vi "Read_binary_data.vi"() -> (0 "Analogue Frequency Hz":dbl format="%.2f", 1 "PWA Binary":i16[][](array[numeric]), 2 "Analogue Binary":i16[][](array[numeric])=[[142, 132, 123, 114, 103, 93, 84, 74, 65, 56, 49, 42, 35, 30, 27, 24, 23, 22, 24, 26, 30, 35, 41, 48, 56, 65, 73, 82, 93, 102, 112, 122, 132, 141, 149, 156, 164, 169, 173, 177, 180, 181, 181, 179, 176, 171, 167, 160, 153, 145, 137, 128, 118, 108, 98, 88, 79, 69, 61, 52, 45, 38, 33, 28, 25, 23, 22, 23, 25, 29, 32, 39, 45, 52, 60, 69, 78, 88, 97, 108, 118, 127, 136, 145, 153, 160, 166, 171, 176, 179, 180, 181, 180, 178, 174, 169, 164, 157, 149, 141]], 3 "PWA Frequency Hz":dbl format="%.2f", 4 "LDA Binary output":u16[][](array[numeric])=[[142, 132, 123, 114, 103, 93, 84, 74, 65, 56, 49, 42, 35, 30, 27, 24, 23, 22, 24, 26, 30, 35, 41, 48, 56, 65, 73, 82, 93, 102, 112, 122, 132, 141, 149, 156, 164, 169, 173, 177, 180, 181, 181, 179, 176, 171, 167, 160, 153, 145, 137, 128, 118, 108, 98, 88, 79, 69, 61, 52, 45, 38, 33, 28, 25, 23, 22, 23, 25, 29, 32, 39, 45, 52, 60, 69, 78, 88, 97, 108, 118, 127, 136, 145, 153, 160, 166, 171, 176, 179, 180, 181, 180, 178, 174, 169, 164, 157, 149, 141]], 5 "EOF?":bool, 6 "Block Header":string)   [LabVIEW 2010]
uses:
  Globals/Meas_global.vi
  Globals/LDA_meas_global_1.vi
panel:
  out "string":string
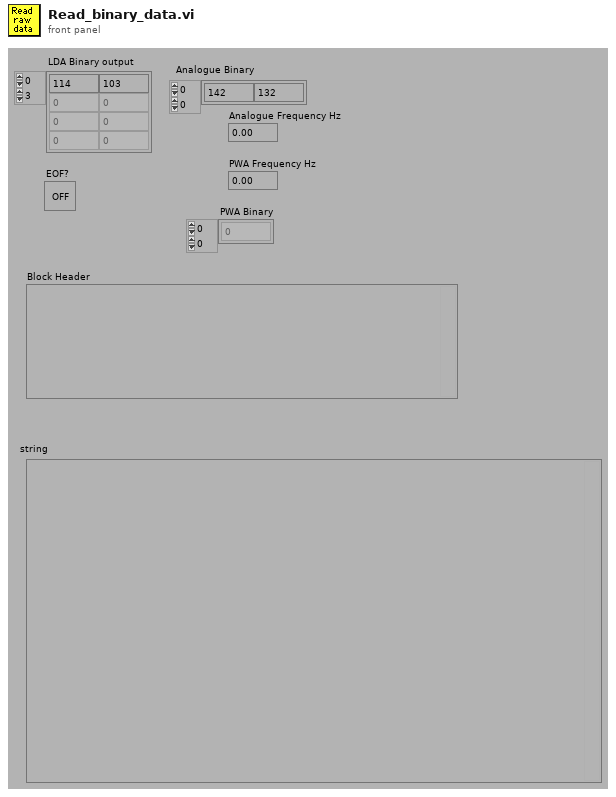
[diagram p1: front panel]
types:
  T1 = enum16{"read/write", "read-only", "write-only", "write-only (truncate)"}
  T2 = typedef "Ch_and_Spans.ctl" = cluster{"high limit (10V)":sgl, "low limit (-10V)":sgl, "Ch No":i16, "Var name":string, "Use Latest Calib":bool}
  T3 = typedef "BSA_Type.ctl" = enum16{"57N11", "BSA F60"}
  T4 = typedef "PWA_Data.ctl" = enum16{"No PWA Data", "One Ch PWA"}
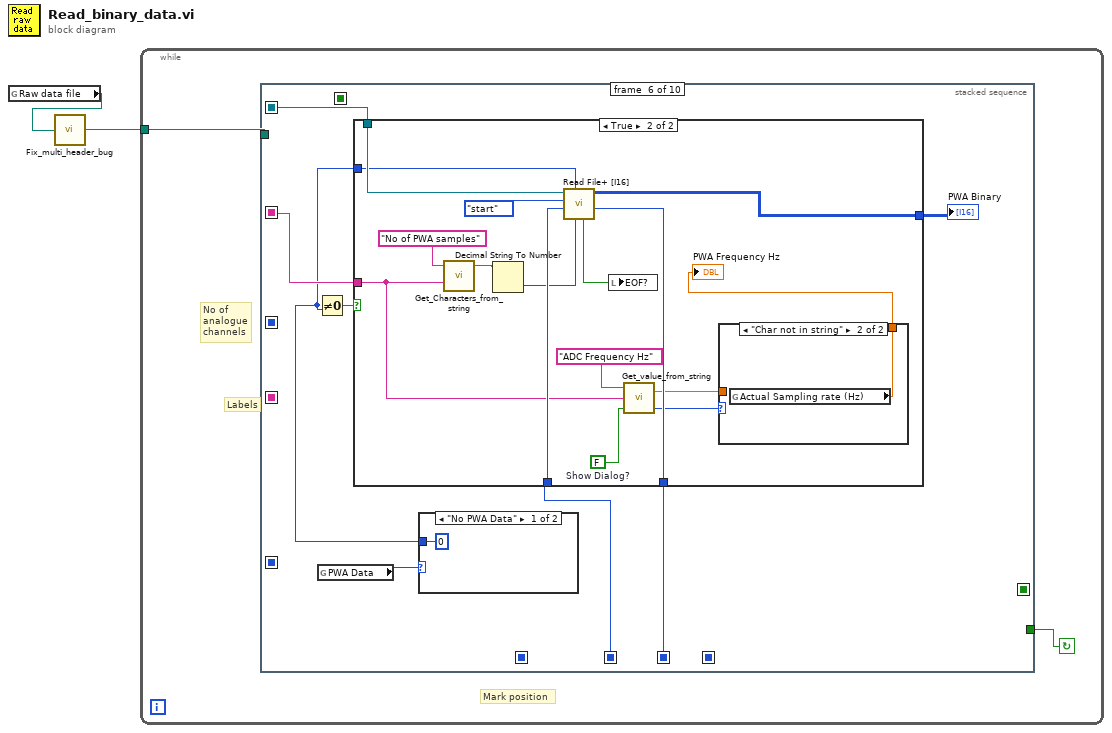
[diagram p0: block diagram]
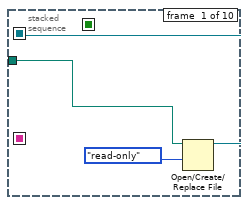
[diagram p2: hidden frame]
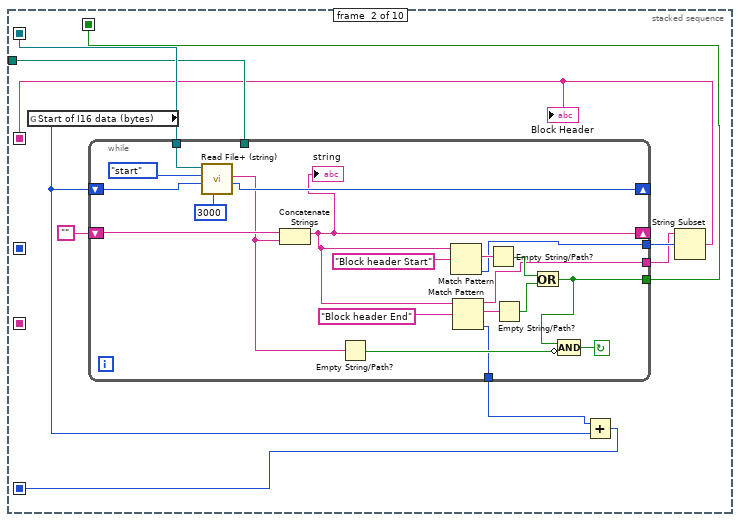
[diagram p3: hidden frame]
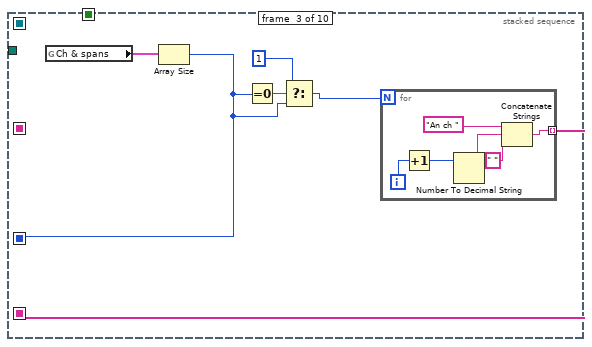
[diagram p4: hidden frame]
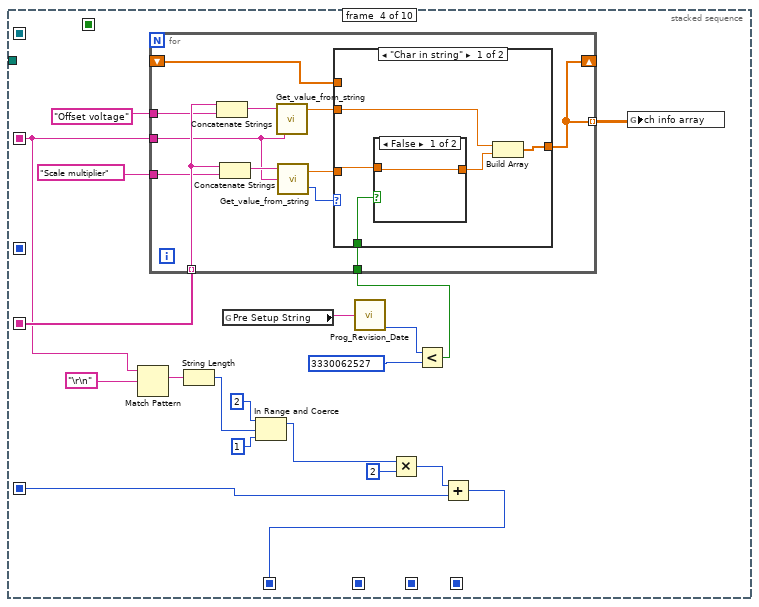
[diagram p5: hidden frame]
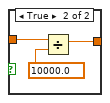
[diagram p6: hidden frame]
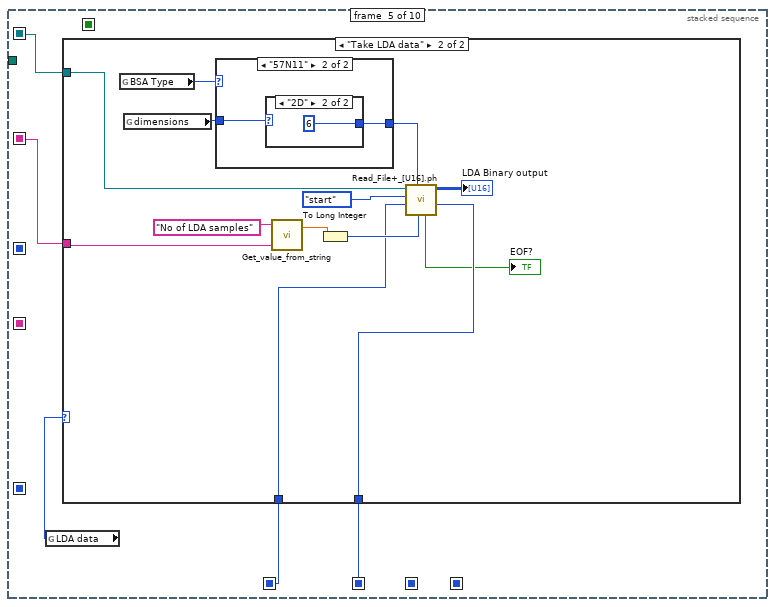
[diagram p8: hidden frame]
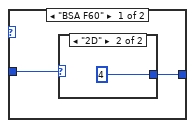
[diagram p10: hidden frame]
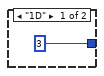
[diagram p11: hidden frame]
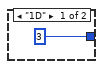
[diagram p12: hidden frame]
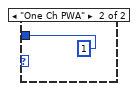
[diagram p13: hidden frame]
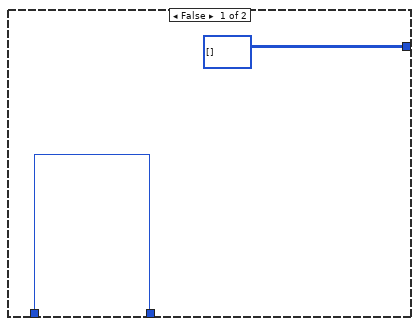
[diagram p14: hidden frame]
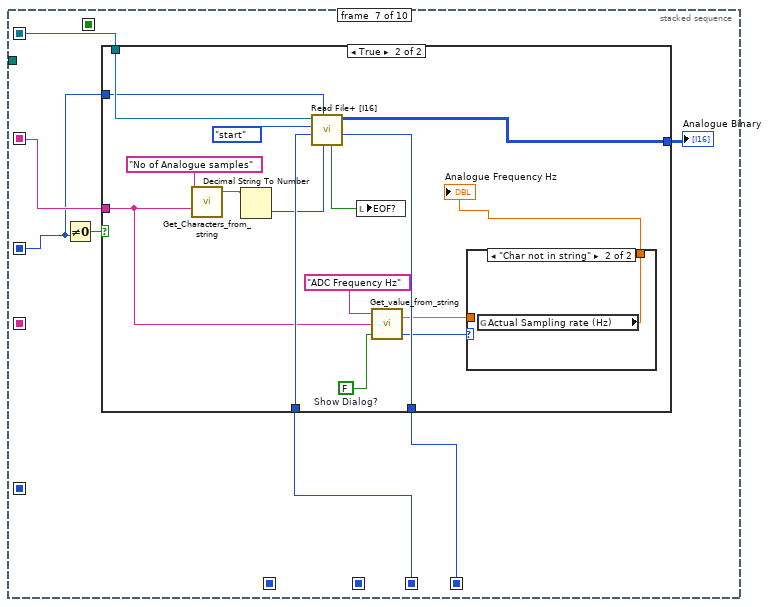
[diagram p16: hidden frame]
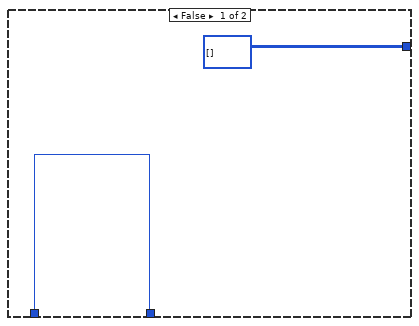
[diagram p17: hidden frame]
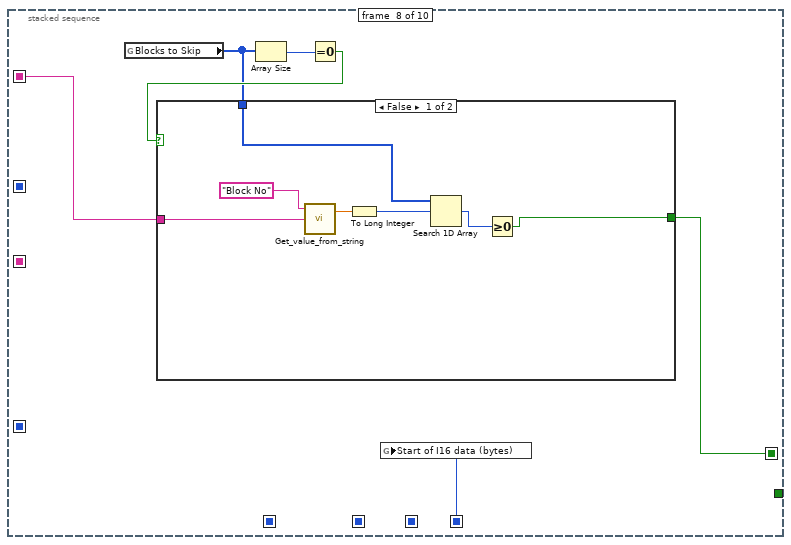
[diagram p19: hidden frame]
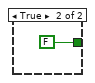
[diagram p20: hidden frame]
diagram:
  n1 = global read "Meas_global.vi" "Raw data file"() -> (w2:path)
  n2 = call "Fix_multi_header_bug.vi"("Raw data File to Read"=w2) -> ("Raw data File to Read Out"=w1:path)
  n3 = while {
    tunnel: w1 -> [w4]
    stop <- w3 continue-if-true
    # "Mark position"
    # "Labels"
    # "No of\nanalogue\nchannels"
    n4 = stacked-sequence {
      seq-local: [w6 _ _ _ _ _ _ _ _ _] -> [_ w17 _ _ w91 w122 w153 _ w194 w213]
      seq-local: [_ w8 _ _ _ _ _ _ _ _] -> [_ _ _ w55 w94 w125 w154 w178 _ _]
      seq-local: [_ _ w40 _ _ _ _ _ _ _] -> [_ _ _ _ _ _ w151 _ _ _]
      seq-local: [_ _ w42 _ _ _ _ _ _ _] -> [_ _ _ w67 _ _ _ _ _ _]
      seq-local: [_ _ _ w64 _ _ _ _ _ _] -> [_ _ _ _ w93 _ _ _ _ _]
      seq-local: [_ _ _ _ w92 _ _ _ _ _] -> [_ _ _ _ _ w124 _ _ _ _]
      seq-local: [_ _ _ _ _ w123 _ _ _ _] -> [_ _ _ _ _ _ w149 _ _ _]
      seq-local: [_ w13 _ _ _ _ _ _ _ _] -> [_ _ _ _ _ _ _ _ _ w214]
      seq-local: [_ w12 _ _ _ _ _ _ _ _] -> [_ _ _ w65 _ _ _ _ _ _]
      seq-local: [_ _ _ _ _ _ _ w176 _ _] -> [_ _ _ _ _ _ _ _ w192 _]
      seq-local: [_ _ _ _ _ _ w148 _ _ _] -> [_ _ _ _ _ _ _ w175 w189 _]
      tunnel: w4 -> [w5 w16 _ _ _ _ _ _ _ w215]
      tunnel: [_ _ _ _ _ _ _ _ w190 _] -> w3
      frame #0 {
        n5 = Open/Create/Replace File(file path (use dialog)=w5, access (0:read/write)=T1."read-only" ("open mode (0)")) -> (refnum out=w6:refnum<file>)  [unwired: 1 in, 5 out]
      }
      frame #1 {
        n6 = global read "Meas_global.vi" "Start of I16 data (bytes)"() -> (w14:i32)
        n7 = while {
          tunnel: [w22] -> w11
          tunnel: [w23] -> w13
          shift-left: "" -> [w26]
          shift-right: [w19] -> _
          tunnel: w16 -> [_]
          tunnel: w17 -> [w35]
          shift-left: w14 -> [w29]
          shift-right: [w34] -> _
          tunnel: [w21] -> w9
          tunnel: [w18] -> w10
          stop <- w30 continue-if-true
          n8 = call <vilib>:"Read File+ (string).vi"("count"=3000, "pos offset (bytes:0)"=w29, "pos mode (rel. to current:2)"=enum16{"start", "end", "current"}."start", "refnum"=w35) -> ("mark after read (bytes)"=w34:i32, "string"=w20:string)  [unwired: 1 in, 5 out]
          n9 = Concatenate Strings(w26, w20) -> (w19:string)
          "string" <- w19
          n10 = Empty String/Path?(string/path=w20) -> (empty?=w31:bool)
          n11 = Match Pattern(string=w19, regular expression="Block header Start") -> (match substring=w28:string, offset past match=w18:i32)  [unwired: 3 out]
          n12 = Match Pattern(string=w19, regular expression="Block header End") -> (before substring=w21:string, match substring=w36:string, offset past match=w22:i32)  [unwired: 2 out]
          n13 = Empty String/Path?(string/path=w28) -> (empty?=w25:bool)
          n14 = Empty String/Path?(string/path=w36) -> (empty?=w24:bool)
          n15 = Or(x=w25, y=w24) -> (x .or. y?=w23:bool)
          n16 = Compound Arithmetic op=AND(w23, invert w31) -> (w30:bool)
        }
        n17 = Add(x=w11, y=w14) -> (x+y=w12:i32)
        n18 = String Subset(string=w9, offset (0)=w10) -> (substring=w8:string)  [unwired: 1 out]
        "Block Header" <- w8
      }
      frame #2 {
        n19 = global read "Meas_global.vi" "Ch & spans"() -> (w43:T2[])
        n20 = Array Size(array=w43) -> (size(s)=w40:i32)
        n21 = Equal To 0?(x=w40) -> (x = 0?=w41:bool)
        n22 = Select(t=1, s=w41, f=w40) -> (s? t:f=w38:i32)
        n23 = for {
          N: w38 -> [_]
          tunnel: [w45] -> w42 mode=indexing
          i -> [w47]
          n24 = Increment(x=w47) -> (x+1=w46:i32)
          n25 = Number To Decimal String(number=w46) -> (decimal integer string=w49:string)  [unwired: 1 out]
          n26 = Concatenate Strings("An ch ", w49, " ") -> (w45:string)
        }
      }
      frame #3 {
        n27 = Match Pattern(string=w55, regular expression="\r\n") -> (match substring=w54:string)  [unwired: 4 out]
        n28 = String Length(string=w54) -> (length=w53:i32)
        n29 = global read "Meas_global.vi" "Pre Setup String"() -> (w59:string)
        n30 = In Range and Coerce(upper limit=2, x=w53, lower limit=1) -> (coerced(x)=w52:i32)  [unwired: 1 out]
        n31 = call "Prog_Revision_Date.vi"("Input string"=w59) -> ("Revision time (s)"=w60:u32)  [unwired: 4 out]
        n32 = Multiply(x=w52, y=2) -> (x*y=w61:i32)
        n33 = Less?(x=w60, y=u32 3330062527 ("unsigned 32bit integer")) -> (x < y?=w57:bool)
        n34 = for {
          tunnel: w67 -> [w80] mode=indexing
          tunnel: "Scale multiplier" -> [w79]
          tunnel: "Offset voltage" -> [w78]
          tunnel: w55 -> [w75]
          tunnel: [w71] -> w68 mode=indexing
          shift-right: [w71] -> _
          shift-left: _ -> [w72]
          tunnel: w57 -> [w69]
          n35 = Concatenate Strings(w80, w78) -> (w77:string)
          n36 = Concatenate Strings(w80, w79) -> (w76:string)
          n37 = call "Get_value_from_string.vi"("Input string"=w75, "Variable name"=w77) -> ("Value"=w73:dbl)  [unwired: 1 in, 1 out]
          n38 = call "Get_value_from_string.vi"("Input string"=w75, "Variable name"=w76) -> ("Status"=w70:enum16{"Char in string", "Char not in string"}, "Value"=w74:dbl)  [unwired: 1 in]
          n39 = case shown="\"Char in string\"" w70 {
            tunnel: w74 -> [w85 _]
            tunnel: w73 -> [w84 _]
            tunnel: [w82 w90] -> w71
            tunnel: w72 -> [_ w90]
            tunnel: w69 -> [w81 _]
            frame "Char in string" {
              n40 = case shown="False" w81 {
                tunnel: w85 -> [w86 w89]
                tunnel: [w86 w87] -> w83
                frame False {
                }
                frame True {
                  n41 = Divide(x=w89, y=10000.0) -> (x/y=w87:dbl)
                }
              }
              n42 = Build Array(w84, w83) -> (w82:dbl[])
            }
            frame "Char not in string" {
            }
          }
        }
        n43 = Add(x=w61, y=w65) -> (x+y=w64:i32)
        n44 = global write "Meas_global.vi" "ch info array"(w68) -> ()
      }
      frame #4 {
        n45 = global read "Meas_global.vi" "LDA data"() -> (w95:enum16{"No LDA data", "Take LDA data"})
        n46 = case shown="\"Take LDA data\"" w95 {
          tunnel: w94 -> [_ w109]
          tunnel: w93 -> [w96 w97]
          tunnel: [w96 w107] -> w92
          tunnel: w91 -> [_ w108]
          frame "No LDA data" {
          }
          frame "Take LDA data" {
            n47 = global read "LDA_meas_global_1.vi" "BSA Type"() -> (w99:T3)
            n48 = global read "Meas_global.vi" "dimensions"() -> (w100:enum16{"1D", "2D"})
            n49 = case shown="\"57N11\"" w99 {
              tunnel: w100 -> [w111 w115]
              tunnel: [w110 w114] -> w98
              frame "BSA F60" {
                n50 = case shown="\"2D\"" w111 {
                  tunnel: [3 4] -> w110
                  frame "1D" {
                  }
                  frame "2D" {
                  }
                }
              }
              frame "57N11" {
                n51 = case shown="\"2D\"" w115 {
                  tunnel: [3 6] -> w114
                  frame "1D" {
                  }
                  frame "2D" {
                  }
                }
              }
            }
            n52 = call "Get_value_from_string.vi"("Input string"=w109, "Variable name"="No of LDA samples") -> ("Value"=w105:dbl)  [unwired: 1 in, 1 out]
            n53 = To Long Integer(number=w105) -> (32bit integer=w103:i32)
            n54 = call "Read_File+_[U16].ph.vi"("2D number of columns/1D count"=w103, "2D number of rows"=w98, "pos offset (bytes:0)"=w97, "pos mode (rel. to current:2)"=enum16{"start", "end", "current"}."start", "refnum"=w108) -> ("mark after read (bytes)"=w107:i32, "2D data"=→"LDA Binary output":u16[][], "EOF?"=→"EOF?":bool)  [unwired: 1 in, 3 out]
          }
        }
      }
      frame #5 {
        n55 = global read "Meas_global.vi" "PWA Data"() -> (w120:T4)
        n56 = case shown="\"No PWA Data\"" w120 {
          tunnel: [0 1] -> w119
          frame "No PWA Data" {
          }
          frame "One Ch PWA" {
          }
        }
        n57 = Not Equal To 0?(x=w119) -> (x != 0?=w121:bool)
        n58 = case shown="True" w121 {
          tunnel: w125 -> [_ w133]
          tunnel: w124 -> [w129 w138]
          tunnel: [w129 w140] -> w123
          tunnel: w122 -> [_ w144]
          tunnel: w119 -> [_ w143]
          tunnel: [i16[][] [] ("2D array") w139] -> w118
          frame False {
          }
          frame True {
            w134 = FALSE  # Show Dialog?
            n59 = call "Get_Characters_from_string.vi"("Input string"=w133, "Variable name"="No of PWA samples") -> ("Value"=w137:string)  [unwired: 1 in, 1 out]
            n60 = Decimal String To Number(string=w137) -> (number=w136:i32)  [unwired: 3 out]
            n61 = call <vilib>:"Read File+ [I16].vi"("2D number of columns/1D count"=w136, "2D number of rows"=w143, "pos offset (bytes:0)"=w138, "pos mode (rel. to current:2)"=enum16{"start", "end", "current"}."start", "refnum"=w144) -> ("mark after read (bytes)"=w140:i32, "2D data"=w139:i16[][], "EOF?"=w141:bool)  [unwired: 1 in, 3 out]
            n62 = local write "EOF?"(w141) -> ()
            n63 = call "Get_value_from_string.vi"("Show Dialog?"=w134, "Input string"=w133, "Variable name"="ADC Frequency Hz") -> ("Status"=w132:enum16{"Char in string", "Char not in string"}, "Value"=w131:dbl)
            n64 = case shown="\"Char not in string\"" w132 {
              tunnel: w131 -> [w146 _]
              tunnel: [w146 w147] -> w130
              frame "Char in string" {
              }
              frame "Char not in string" {
                n65 = global read "Meas_global.vi" "Actual Sampling rate (Hz)"() -> (w147:dbl)
              }
            }
            "PWA Frequency Hz" <- w130
          }
        }
        "PWA Binary" <- w118
      }
      frame #6 {
        n66 = Not Equal To 0?(x=w151) -> (x != 0?=w152:bool)
        n67 = case shown="True" w152 {
          tunnel: w154 -> [_ w160]
          tunnel: w149 -> [w156 w165]
          tunnel: [w156 w167] -> w148
          tunnel: w153 -> [_ w171]
          tunnel: w151 -> [_ w170]
          tunnel: [i16[][] [] ("2D array") w166] -> w150
          frame False {
          }
          frame True {
            w161 = FALSE  # Show Dialog?
            n68 = call "Get_Characters_from_string.vi"("Input string"=w160, "Variable name"="No of Analogue samples") -> ("Value"=w164:string)  [unwired: 1 in, 1 out]
            n69 = Decimal String To Number(string=w164) -> (number=w163:i32)  [unwired: 3 out]
            n70 = call <vilib>:"Read File+ [I16].vi"("2D number of columns/1D count"=w163, "2D number of rows"=w170, "pos offset (bytes:0)"=w165, "pos mode (rel. to current:2)"=enum16{"start", "end", "current"}."start", "refnum"=w171) -> ("mark after read (bytes)"=w167:i32, "2D data"=w166:i16[][], "EOF?"=w168:bool)  [unwired: 1 in, 3 out]
            n71 = local write "EOF?"(w168) -> ()
            n72 = call "Get_value_from_string.vi"("Show Dialog?"=w161, "Input string"=w160, "Variable name"="ADC Frequency Hz") -> ("Status"=w159:enum16{"Char in string", "Char not in string"}, "Value"=w158:dbl)
            n73 = case shown="\"Char not in string\"" w159 {
              tunnel: w158 -> [w173 _]
              tunnel: [w173 w174] -> w157
              frame "Char in string" {
              }
              frame "Char not in string" {
                n74 = global read "Meas_global.vi" "Actual Sampling rate (Hz)"() -> (w174:dbl)
              }
            }
            "Analogue Frequency Hz" <- w157
          }
        }
        "Analogue Binary" <- w150
      }
      frame #7 {
        n75 = global read "Meas_global.vi" "Blocks to Skip"() -> (w177:i32[])
        n76 = Array Size(array=w177) -> (size(s)=w180:i32)
        n77 = Equal To 0?(x=w180) -> (x = 0?=w179:bool)
        n78 = case shown="False" w179 {
          tunnel: w178 -> [w186 _]
          tunnel: w177 -> [w183 _]
          tunnel: [w181 FALSE] -> w176
          frame False {
            n79 = call "Get_value_from_string.vi"("Input string"=w186, "Variable name"="Block No") -> ("Value"=w185:dbl)  [unwired: 1 in, 1 out]
            n80 = To Long Integer(number=w185) -> (32bit integer=w184:i32)
            n81 = Search 1D Array(1D array=w183, element=w184) -> (index of element=w182:i32)  [unwired: 1 out]
            n82 = Greater Or Equal To 0?(x=w182) -> (x >= 0?=w181:bool)
          }
          frame True {
          }
        }
        n83 = global write "Meas_global.vi" "Start of I16 data (bytes)"(w175) -> ()
      }
      frame #8 {
        n84 = local read "EOF?"() -> (w193:bool)
        n85 = case shown="False" w193 {
          tunnel: w189 -> [w197 _]
          tunnel: w194 -> [w196 _]
          tunnel: [w195 w211] -> w191
          tunnel: w193 -> [_ w211]
          frame False {
            n86 = while {
              tunnel: [w201] -> w195
              tunnel: w196 -> [w208]
              shift-left: w197 -> [w203]
              shift-right: [w204] -> _
              stop <- w199 continue-if-true
              n87 = call <vilib>:"Read File+ (string).vi"("count"=3000, "pos offset (bytes:0)"=w203, "pos mode (rel. to current:2)"=enum16{"start", "end", "current"}."start", "refnum"=w208) -> ("error out"=w202:errorcluster, "mark after read (bytes)"=w204:i32, "string"=w205:string, "EOF?"=w198:bool)  [unwired: 1 in, 3 out]
              n88 = Unbundle By Name(w202) -> ("status"=w200:bool)
              n89 = Match Pattern(string=w205, regular expression="Block header") -> (match substring=w209:string)  [unwired: 4 out]
              n90 = Empty String/Path?(string/path=w209) -> (empty?=w201:bool)
              n91 = Compound Arithmetic op=AND(w201, invert w200, invert w198) -> (w199:bool)
            }
          }
          frame True {
          }
        }
        n92 = local write "EOF?"(w191) -> ()
        n93 = Compound Arithmetic op=AND(w192, invert w191) -> (w190:bool)
      }
      frame #9 {
        n94 = Close File(refnum=w213) -> (error out=w212:errorcluster)  [unwired: 1 in, 1 out]
        n95 = case shown="False" w214 {
          tunnel: w215 -> [w218 _]
          tunnel: w212 -> [w216 _]
          frame False {
            n96 = call "Add_filename_to_err_message.vi"("error in (no error)"=w216, "Path"=w218) -> ("error out"=w219:errorcluster)
            n97 = call "EnFlo_Error_Handler.vi"("error in (no error)"=w219, "Dialog Box (T)"=TRUE) -> ()  [unwired: 1 in, 3 out]
          }
          frame True {
            w223 = FALSE  # Dialog Box
            n98 = Bundle By Name(cluster=errorcluster {"status"=FALSE, "code"=0, "source"=""} ("error in (no error)"), "status"=TRUE ("Bundle Element"), "source"="The block header was not found in the file" ("Bundle Element")) -> (w224:errorcluster)
            n99 = call "EnFlo_Error_Handler.vi"("error in (no error)"=w224, "Error Type"="Raw Data File Error", "Dialog Box (T)"=w223) -> ()  [unwired: 3 out]
          }
        }
      }
    }
  }
